vi "Boolean Operations.vi"() -> ()   [LabVIEW 2020]
panel:
  out "Boolean NOT OR":bool
  out "Boolean implies":bool
  out "Boolean NOT XOR":bool
  out "Boolean NOT AND":bool
  out "Boolean NOT":bool
  out "Boolean XOR":bool
  out "Boolean OR":bool
  out "Boolean AND":bool
  in  "B":bool
  in  "A":bool
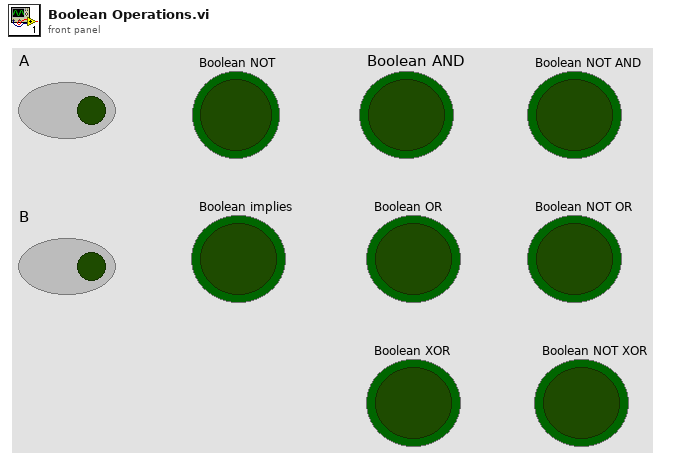
[diagram p1: front panel]
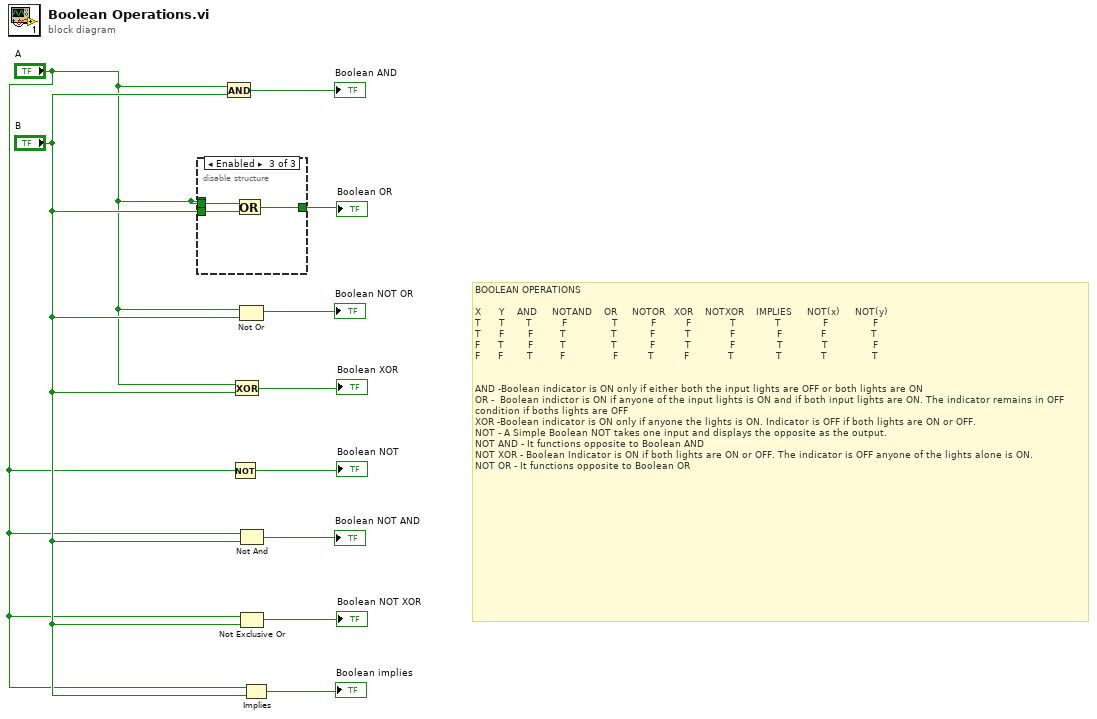
[diagram p0: block diagram]
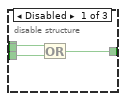
[diagram p2: hidden frame]
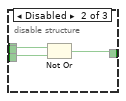
[diagram p3: hidden frame]
diagram:
  # "BOOLEAN OPERATIONS\n \nX      Y    AND     NOTAND    OR     NOTOR   XOR    NOTXOR    IMPLIES     NOT(x)     NOT(y)\nT      T       T          F               T           F          F             T             T              F               F   \nT      F        F         T               T           F          T             F              F             F               T\nF      T        F         T               T           F          T             F              T             T               F\nF      F        T         F                F          T          F             T              T             T               T\n\n\nAND -Boolean indicator is ON only if either both the input lights are OFF or both lights are ON\nOR -  Boolean indictor is ON if anyone of the input lights is ON and if both input lights are ON. The indicator remains in OFF condition if boths lights are OFF\nXOR -Boolean indicator is ON only if anyone the lights is ON. Indicator is OFF if both lights are ON or OFF.\nNOT - A Simple Boolean NOT takes one input and displays the opposite as the output.\nNOT AND - It functions opposite to Boolean AND \nNOT XOR - Boolean Indicator is ON if both lights are ON or OFF. The indicator is OFF anyone of the lights alone is ON.\nNOT OR - It functions opposite to Boolean OR"
  n1 = disable-structure shown="Enabled" {
    disable-tunnel: [w13 w16 w17] -> w9
    disable-tunnel: "A" -> [w12 w15 _]
    disable-tunnel: "A" -> [_ _ w19]
    disable-tunnel: "B" -> [w11 w14 w18]
    frame Disabled {
      n2 = Or(x=w12, y=w11) -> (x .or. y?=w13:bool)
    }
    frame Disabled {
      n3 = Not Or(1:w14, 2:w15) -> (0:w16:bool)
    }
    frame Enabled {
      n4 = Or(x=w19, y=w18) -> (x .or. y?=w17:bool)
    }
  }
  "Boolean OR" <- w9
  n5 = And(x="A", y="B") -> (x .and. y?=→"Boolean AND":bool)
  n6 = Not(x="A") -> (.not. x?=→"Boolean NOT":bool)
  n7 = Exclusive Or(1:"B", 2:"A") -> (0:→"Boolean XOR":bool)
  n8 = Not Or(1:"B", 2:"A") -> (0:→"Boolean NOT OR":bool)
  n9 = Not And(1:"B", 2:"A") -> (0:→"Boolean NOT AND":bool)
  n10 = Not Exclusive Or(1:"B", 2:"A") -> (0:→"Boolean NOT XOR":bool)
  n11 = Implies(1:"B", 2:"A") -> (0:→"Boolean implies":bool)
